vi "Filter.vi"() -> ()   [LabVIEW 2011]
uses:
  <vilib>/Analysis/3filter.llb/Filter Passband Type.ctl
  <vilib>/measure/maspectr.llb/FFT Spectrum (Mag-Phase) for 1 Chan.vi
  <vilib>/Analysis/3filter.llb/Chebyshev Filter (DBL).vi
  <vilib>/measure/NI_MABase.lvlib
  <vilib>/Analysis/NI_AALBase.lvlib
  <vilib>/measure/NI_MAPro.lvlib
panel:
  in  "signal type":T1(ring)=enum."Square Wave"
  in  "Cut-off Frequency - High":dbl(knob)=10.0 scale=0.0..10.0
  in  "Cut-off Frequency - Low":dbl(knob)=5.0 scale=0.0..10.0
  in  "Frequency":dbl(knob)=10.0 scale=0.0..10.0
  in  "stop":bool
  out "FFT":cluster{"f0":dbl, "df":dbl, "magnitude":dbl[]}(graph)
  out "Source FFT":cluster{"f0":dbl, "df":dbl, "magnitude":dbl[]}(graph)
  out "Filtered":waveform(dbl)(graph)
  out "Source Waveform":waveform(dbl)(graph)
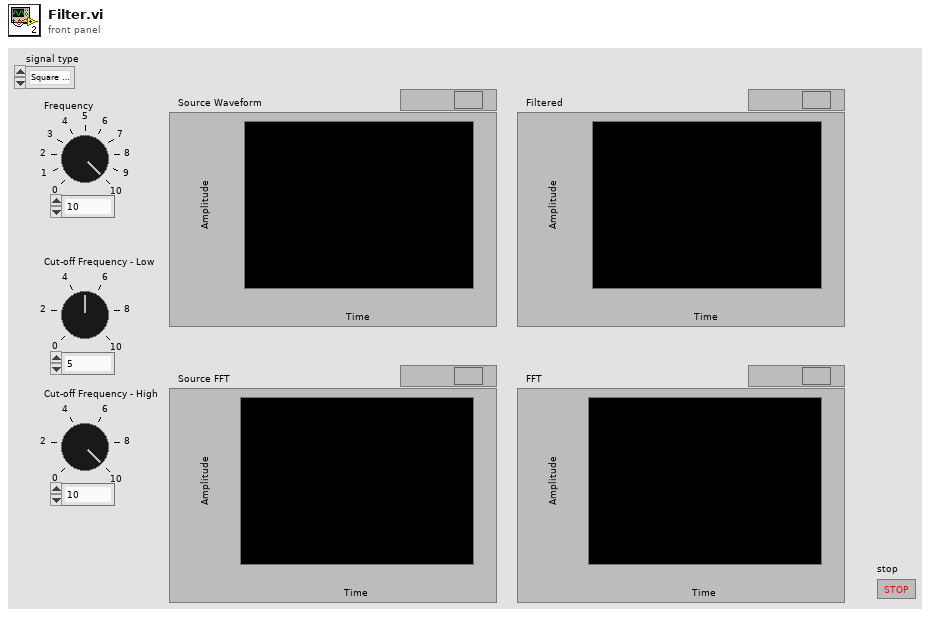
[diagram p1: front panel]
types:
  T1 = enum16{"Sine Wave", "Triangle Wave", "Square Wave", "Sawtooth Wave"}
  T2 = typedef "NI_AALBase.lvlib/Filter Passband Type.ctl" = enum32{"Lowpass", "Highpass", "Bandpass", "Bandstop"}
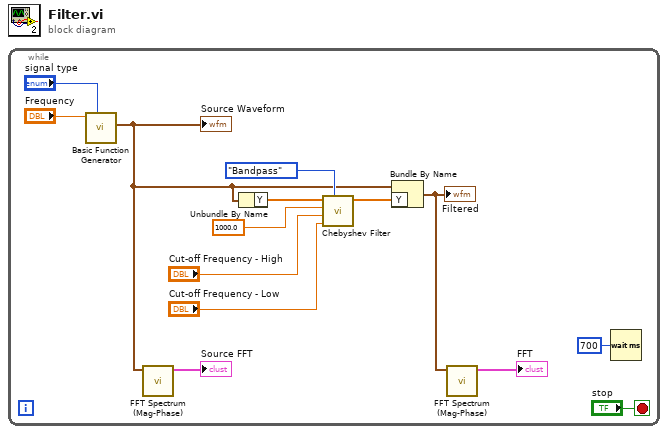
[diagram p0: block diagram]
diagram:
  n1 = while {
    stop <- "stop" stop-if-true
    n2 = call <vilib>:"Basic Function Generator.vi"("signal type"="signal type", "frequency"="Frequency") -> ("signal out"=w5:waveform(dbl))  [unwired: 7 in, 2 out]
    "Source Waveform" <- w5
    n3 = call-poly <vilib>:"FFT Spectrum (Mag-Phase).vi"("time signal"=w5) -> ("magnitude"=→"Source FFT":cluster{"f0":dbl, "df":dbl, "magnitude":dbl[]})  [unwired: 6 in, 4 out]
    n4 = Unbundle By Name(w5) -> ("Y"=w12:dbl[])
    n5 = call-poly <vilib>:"Chebyshev Filter.vi"("filter type"=Filter_Passband_Type."Bandpass", "low cutoff freq: fl"="Cut-off Frequency - Low", "high cutoff freq: fh"="Cut-off Frequency - High", "sampling freq: fs"=1000.0, "X"=w12) -> ("Filtered X"=w11:dbl[])  [unwired: 5 in, 1 out]
    n6 = Bundle By Name(cluster=w5, "Y"=w11) -> (w3:waveform(dbl))
    "Filtered" <- w3
    n7 = call-poly <vilib>:"FFT Spectrum (Mag-Phase).vi"("time signal"=w3) -> ("magnitude"=→"FFT":cluster{"f0":dbl, "df":dbl, "magnitude":dbl[]})  [unwired: 6 in, 4 out]
    n8 = Wait (ms)(milliseconds to wait=u32 700) -> ()  [unwired: 1 out]
  }
